vi "SOUR_POW_ATT_AUTO_OFF.vi"(0 "VISA IN":refnum<visa-resource-name>, 1 "Port number":i32, 2 "ATTN":i32, 3 "AUTO ON/OFF":bool, 5 "error in":errorcluster, 7 "Channel":i32) -> (14 "VISA Out":refnum<visa-resource-name>, 19 "error out":errorcluster)   [LabVIEW 2018, in "PNA-X.lvlib"]
doc: "SOURce:POWer:ATTenuation <num>) sets AUTO OFF. \nParameters \n<cnum> Any existing channel number. If unspecified, value is set to 1. \n<port> Port number of the PNA. If unspecified, value is set to 1.To make settings for \nports that are not simple numbers, use the [src] argument. \n<bool> ON (or 1) - turns coupling ON. The analyzer automatically selects the \nappropriate attenuation level to meet the specified power level. \nOFF (or 0) - turns coupling OFF. Attenuation level must be set using"
uses:
  PNA-X.lvlib
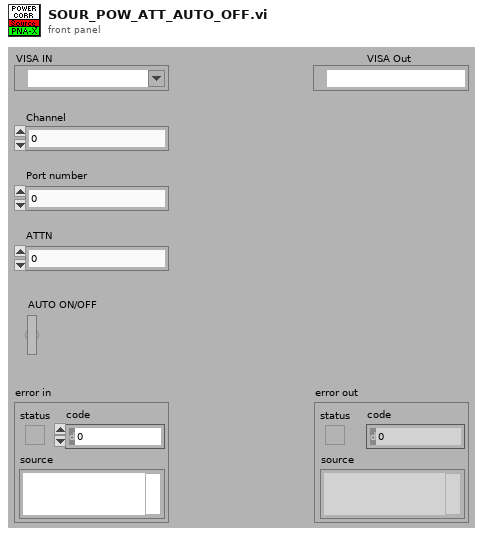
[diagram p1: front panel]
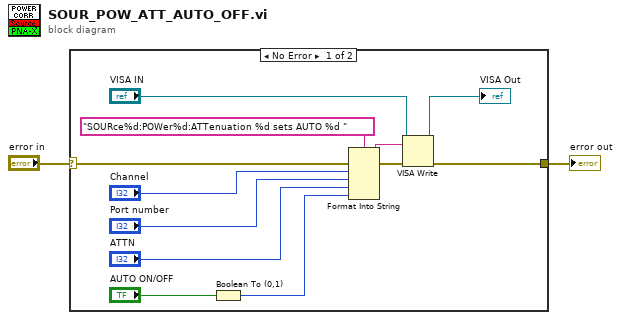
[diagram p0: block diagram]
diagram:
  n1 = case shown="No Error" "error in" {
    selector: "error in" -> [w14 w15]
    tunnel: [w9 w15] -> w1
    frame No Error {
      n2 = Boolean To (0,1)(Boolean="AUTO ON/OFF") -> (0, 1=w3:i16)
      n3 = Format Into String(format string="SOURce%d:POWer%d:ATTenuation %d sets AUTO %d " ("Cmdline"), error in=w14, "Channel", "Port number", "ATTN", w3) -> (resulting string=w12:string, error out=w13:errorcluster)  [unwired: 1 in]
      n4 = VISA Write(VISA resource name="VISA IN", write buffer=w12, error in (no error)=w13) -> (VISA resource name out=→"VISA Out":refnum<visa-resource-name>, error out=w9:errorcluster)  [unwired: 1 out]
    }
    frame Error {
    }
  }
  "error out" <- w1
